vi "Paskevits_Vladislav_gbl1.vi"() -> ()   [LabVIEW 2018]
doc: "This GlobalVariable are working with temperature"
panel:
  out "Temperature":dbl
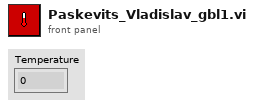
[diagram p1: front panel]
diagram:
